vi "ztscopeM Channel Query.vi"(8 "error in":errorcluster, 10 "Channel":i32(ring) items=["Input Channel 1", "Input Channel 2", "Input Channel 3", "Input Channel 4"], 11 "Instrument Handle In":i32) -> (0 "error out":errorcluster, 2 "State":i32, 3 "Instrument Handle Out":i32)   [LabVIEW 2013]
doc: "Query the state of the selected input channel."
uses:
  ztscopeM.dll
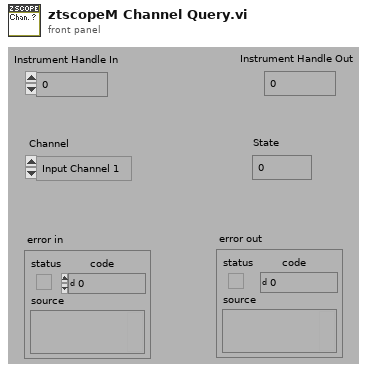
[diagram p1: front panel]
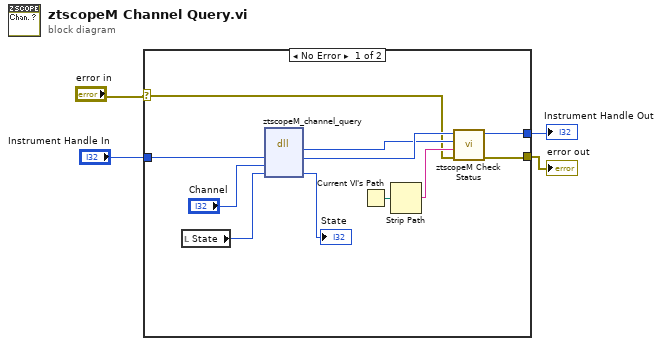
[diagram p0: block diagram]
diagram:
  n1 = case shown="No Error" "error in" {
    selector: "error in" -> [w7 w17]
    tunnel: [w6 w17] -> w1
    tunnel: "Instrument Handle In" -> [w15 w16]
    tunnel: [w5 w16] -> w3
    frame No Error {
      n2 = local read "State"() -> (w13:i32)
      n3 = dll-call lib="C:/Program Files/National Instruments/instr.lib/ztscopem/ztscopeM.dll" fn="ztscopeM_channel_query"("instrumentHandle"=w15, "channel"="Channel", "state"=w13) -> (w8:i32, "instrumentHandle"=w9:i32, "state"=→"State":i32)  [unwired: 4 in, 2 out]
      n4 = Current VI's Path() -> (path=w11:path)
      n5 = Strip Path(path=w11) -> (name=w10:string)  [unwired: 1 out]
      n6 = call "ztscopeM Check Status.vi"("error in"=w7, "name of VI"=w10, "status"=w8, "instrument handle in"=w9) -> ("error out"=w6:errorcluster, "instrument handle out"=w5:i32)  [unwired: 2 in]
    }
    frame Error {
    }
  }
  "Instrument Handle Out" <- w3
  "error out" <- w1
